vi "通用报警记录缓存文件列表.vi"(11 "文件类型（全部）":enum16{"全部报警文件", "剂量率报警文件", "累积剂量报警文件"}(ring)) -> (3 "报警记录文件":path[](array[path]))   [LabVIEW 2017]
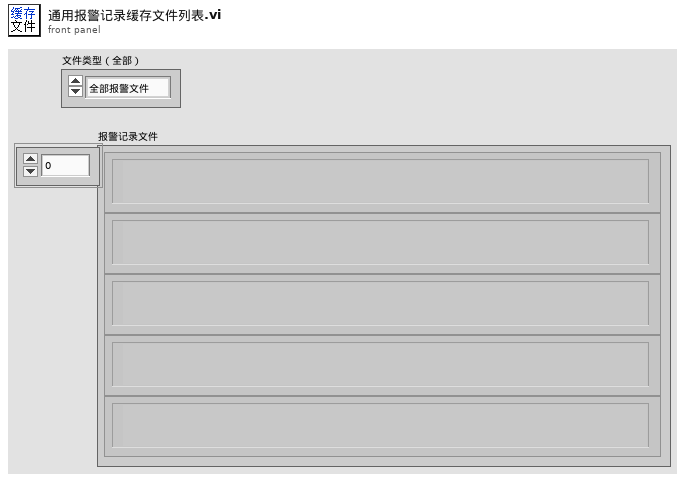
[diagram p1: front panel]
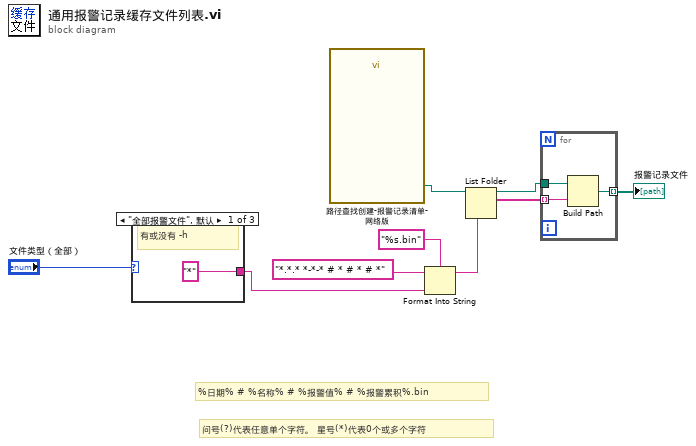
[diagram p0: block diagram]
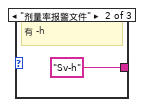
[diagram p2: hidden frame]
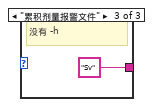
[diagram p3: hidden frame]
diagram:
  # "%日期% # %名称% # %报警值% # %报警累积%.bin"
  # "问号(?)代表任意单个字符。 星号(*)代表0个或多个字符"
  n1 = case shown="\"全部报警文件\", 默认" "文件类型（全部）" {
    tunnel: ["*" ("初始字符串") "Sv-h" ("初始字符串") "Sv" ("初始字符串")] -> w2
    frame "全部报警文件", Default {
      # "有或没有 -h"
    }
    frame "剂量率报警文件" {
      # "有 -h"
    }
    frame "累积剂量报警文件" {
      # "没有 -h"
    }
  }
  n2 = call "路径查找创建-报警记录清单-网络版.vi"() -> ("缓存数据文件夹"=w9:path)  [unwired: 2 in, 13 out]
  n3 = Format Into String(format string="%s.bin" ("格式字符串"), initial string="*.*.* *-*-* # * # * # *" ("初始字符串"), w2) -> (resulting string=w1:string)  [unwired: 1 in, 1 out]
  n4 = List Folder(path=w9, pattern=w1) -> (path out=w8:path, filenames=w7:string[])  [unwired: 2 in, 2 out]
  n5 = for {
    tunnel: w8 -> [w15]
    tunnel: w7 -> [w14] mode=indexing
    tunnel: [w13] -> w6 mode=indexing
    n6 = Build Path(base path=w15, name or relative path=w14) -> (appended path=w13:path)
  }
  "报警记录文件" <- w6
